vi "Change Camera.vi"(8 "error in (no error)":errorcluster, 10 "New Camera":string, 11 "IMAQdx Actor in":refnum<class "IMAQdx Actor.lvclass">) -> (0 "error out":errorcluster, 3 "IMAQdx Actor out":refnum<class "IMAQdx Actor.lvclass">)   [LabVIEW 2020, in "IMAQdx Actor.lvlib" / "IMAQdx Actor.lvclass"]
uses:
  IMAQdx Actor.lvclass
  Camera Actor/Camera Actor/Camera Actor.lvclass
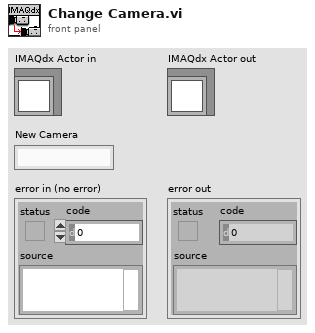
[diagram p1: front panel]
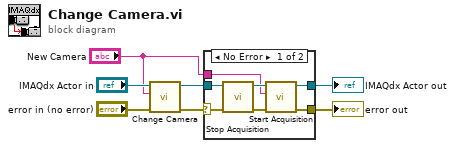
[diagram p0: block diagram]
diagram:
  n1 = call-parent "Change Camera.vi"("error in (no error)"="error in (no error)", "New Camera"="New Camera", "Camera Actor in"="IMAQdx Actor in") -> ("error out"=w1:errorcluster, "Camera Actor out"=w4:refnum<class "IMAQdx Actor.lvclass">)  [unwired: 7 in]
  n2 = case shown="No Error" w1 {
    selector: w1 -> [w8 w15]
    tunnel: w4 -> [w13 w16]
    tunnel: "New Camera" -> [w11 _]
    tunnel: [w10 w16] -> w6
    tunnel: [w9 w15] -> w5
    frame No Error {
      n3 = call-dynamic "Stop Acquisition.vi"("error in (no error)"=w8, "IMAQdx Actor in"=w13) -> ("error out"=w12:errorcluster, "IMAQdx Actor out"=w14:refnum<class "IMAQdx Actor.lvclass">)  [unwired: 8 in]
      n4 = call-dynamic "Start Acquisition.vi"("error in (no error)"=w12, "Camera Name"=w11, "IMAQdx Actor in"=w14) -> ("error out"=w9:errorcluster, "IMAQdx Actor out"=w10:refnum<class "IMAQdx Actor.lvclass">)  [unwired: 7 in]
    }
    frame Error {
    }
  }
  "error out" <- w5
  "IMAQdx Actor out" <- w6
